vi "FlipEye.vi"() -> ()   [LabVIEW 2022 SP3]
panel:
  in  "Boolean":bool
  out "Raw data":i8[][](graph)
  in  "new eye file path":path
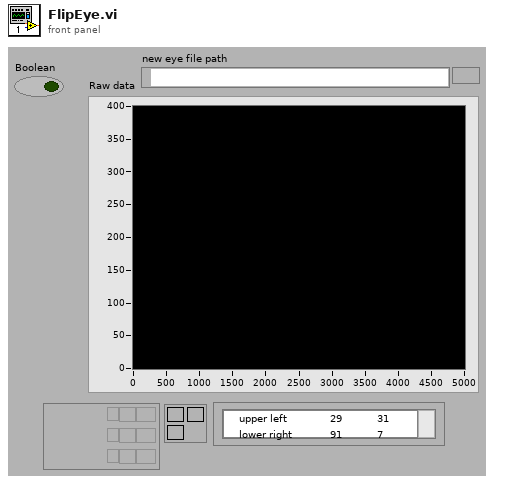
[diagram p1: front panel]
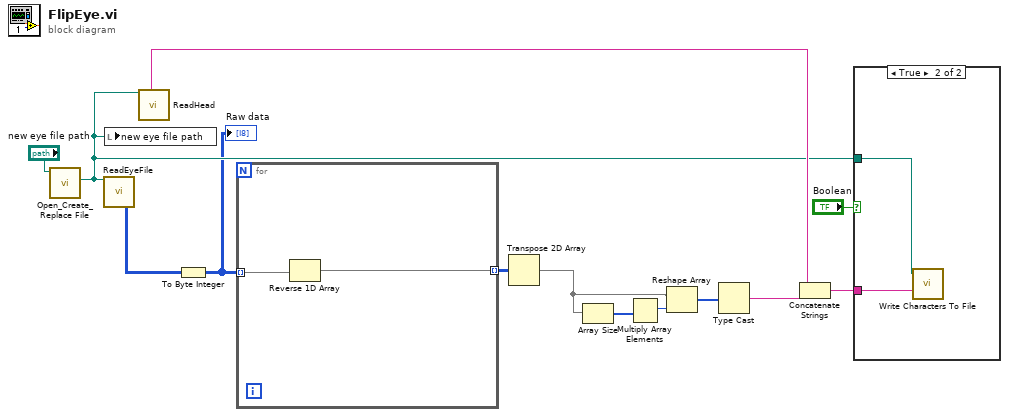
[diagram p0: block diagram]
diagram:
  n1 = call <vilib>:"Open_Create_Replace File.vi"("file path"="new eye file path") -> ("new file path"=w4:path)  [unwired: 5 in, 5 out]
  n2 = call "ReadEyeFile.vi"("new file path"=w4) -> ("2-D data array"=w12:i16[][])  [unwired: 1 in, 17 out]
  n3 = local write "new eye file path"(w4) -> ()
  n4 = call "ReadHead.vi"("new file path"=w4) -> ("whole header"=w7:string)  [unwired: 18 out]
  n5 = To Byte Integer(number=w12) -> (8bit integer=w1:i8[][])
  "Raw data" <- w1
  n6 = for {
    tunnel: w1 -> [w15] mode=indexing
    tunnel: [w14] -> w2 mode=indexing
    n7 = Reverse 1D Array(array=w15) -> (reversed array=w14:i8[])
  }
  n8 = Transpose 2D Array(2D array=w2) -> (transposed array=w5:i8[][])
  n9 = Array Size(array=w5) -> (size(s)=w11:i32[])
  n10 = Multiply Array Elements(1:w11) -> (0:w10:i32)
  n11 = Reshape Array(w5, w10) -> (w9:i8[])
  n12 = Type Cast(x=w9) -> (*(type *) &x=w8:string)  [unwired: 1 out]
  n13 = Concatenate Strings(w7, w8) -> (w6:string)
  n14 = case shown="True" "Boolean" {
    tunnel: w6 -> [_ w17]
    tunnel: w4 -> [_ w16]
    frame False {
    }
    frame True {
      n15 = call <vilib>:"Write Characters To File.vi"("character string"=w17, "file path (dialog if empty)"=w16) -> ()  [unwired: 1 in, 3 out]
    }
  }
